vi "Calculate Efficiency.vi"(9 "output power per channel":dbl[](array[numeric]), 10 "power supply current":dbl, 11 "power supply voltage":dbl) -> (0 "efficiency":dbl, 1 "power loss":dbl, 2 "total output power":dbl, 3 "input power":dbl)   [LabVIEW 2021]
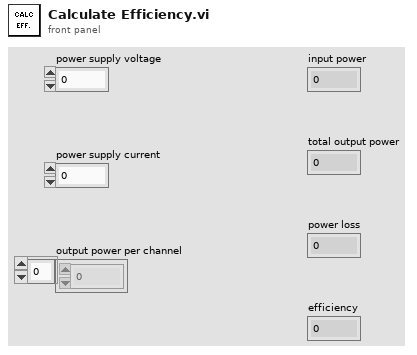
[diagram p1: front panel]
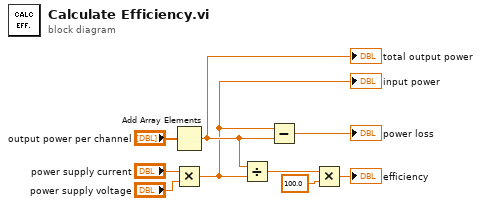
[diagram p0: block diagram]
diagram:
  n1 = Add Array Elements(numeric array="output power per channel") -> (sum=w8:dbl)
  "total output power" <- w8
  n2 = Multiply(x="power supply current", y="power supply voltage") -> (x*y=w5:dbl)
  "input power" <- w5
  n3 = Divide(x=w8, y=w5) -> (x/y=w1:dbl)
  n4 = Subtract(x=w5, y=w8) -> (x-y=→"power loss":dbl)
  n5 = Multiply(x=w1, y=100.0) -> (x*y=→"efficiency":dbl)
